vi "Run 1 home.vi"(11 "EV3 in":T1) -> ()   [LabVIEW 2016]
uses:
  <vilib>/NXT/Subs/LVHSConnector.ctl
  <vilib>/NXT/LegoClasses/BrickReference/BrickReference.lvclass
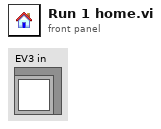
[diagram p1: front panel]
types:
  T1 = typedef "LVHSConnector.ctl" = refnum<class "BrickReference.lvclass">
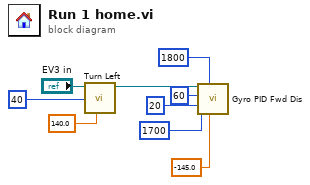
[diagram p0: block diagram]
diagram:
  n1 = call "Turn Left.vi"("Turning angle"=sgl 140.0, "Motor B (right)"=i8 40, "EV3 in"="EV3 in") -> ("EV3 out"=w6:T1)  [unwired: 8 in]
  n2 = call "Gyro PID Fwd Dis.vi"("Target angle"=sgl -145.0, "Threshold to stop"=1800, "Threshold to slow"=1700, "Min. speed"=20, "Max. speed"=60, "EV3 in"=w6) -> ()  [unwired: 5 in, 1 out]
